vi "setParameters.vi"(10 "Parameters":T1, 11 "RaiseM1M3Command in":refnum<class "RaiseM1M3Command.lvclass">) -> (3 "RaiseM1M3Command out":refnum<class "RaiseM1M3Command.lvclass">)   [LabVIEW 2016, in "RaiseM1M3Command.lvclass"]
uses:
  RaiseM1M3Command.lvclass
  DataTypes/Topics/CommandRaiseM1M3.ctl
  DataTypes/Topics/Parts/CommandId.ctl
  RaiseM1M3Command.lvclass/RaiseM1M3Command.ctl
  DataTypes/Topics/M1M3SupportTopics.lvlib
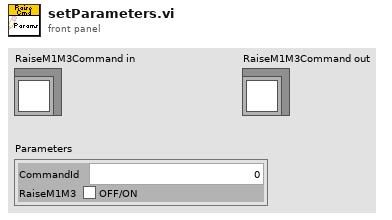
[diagram p1: front panel]
types:
  T1 = typedef "M1M3SupportTopics.lvlib/CommandRaiseM1M3.ctl" = cluster{"CommandId":T2, "RaiseM1M3":bool}
  T2 = typedef "M1M3SupportTopics.lvlib/CommandId.ctl" = i32
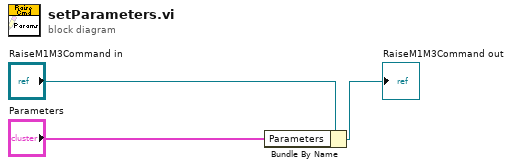
[diagram p0: block diagram]
diagram:
  n1 = Bundle By Name(cluster="RaiseM1M3Command in", "Parameters"="Parameters") -> (→"RaiseM1M3Command out":refnum<class "RaiseM1M3Command.lvclass">)
